vi "Visualize_Results_of_Filtering-1.vi"(7 "[IN] Number of event":i8=2, 8 "error IN":errorcluster, 9 "[IN] Localization Settings":T5 {"[IN] Image Type" items=["Grayscale (U8)", "Grayscale (I16)", "Grayscale (SGL)", "Complex (CSG)", "RGB (U32)", "HSL (U32)", "RGB (U64)", "Grayscale (U16)"]; "[IN] Particle Filter Setups"."Type of particle filter"."Measurement Parameter" items=["Center of Mass X", "Center of Mass Y", "First Pixel X", "First Pixel Y", "Bounding Rect Left", "Bounding Rect Top", "Bounding Rect Right", "Bounding Rect Bottom", "Max Feret Diameter Start X", "Max Feret Diameter Start Y", "Max Feret Diameter End X", "Max Feret Diameter End Y", "Max Horiz. Segment Length Left", "Max Horiz. Segment Length Right", "Max Horiz. Segment Length Row", "-", "Bounding Rect Width", "Bounding Rect Height", "Bounding Rect Diagonal", "Perimeter", "Convex Hull Perimeter", "Holes' Perimeter", "Max Feret Diameter", "Equivalent Ellipse Major Axis", "Equivalent Ellipse Minor Axis", "Equivalent Ellipse Minor Axis (Feret)", "Equivalent Rect Long Side", "Equivalent Rect Short Side", "Equivalent Rect Diagonal", "Equivalent Rect Short Side (Feret)", "Average Horiz. Segment Length", "Average Vert. Segment Length", "Hydraulic Radius", "Waddel Disk Diameter", "-", "Area", "Holes' Area", "Particle & Holes' Area", "Convex Hull Area", "Image Area", "-", "Number of Holes", "Number of Horiz. Segments", "Number of Vert. Segments", "-", "Orientation", "Max Feret Diameter Orientation", "-", "% Area/Image Area", "% Area/(Particle & Holes' Area)", "Ratio of Equivalent Ellipse Axes", "Ratio of Equivalent Rect Sides", "-", "Elongation Factor", "Compactness Factor", "Heywood Circularity Factor", "Type Factor", "-", "Sum X", "Sum Y", "Sum XX", "Sum XY", "Sum YY", "Sum XXX", "Sum XXY", "Sum XYY", "Sum YYY", "-", "Moment of Inertia XX", "Moment of Inertia XY", "Moment of Inertia YY", "Moment of Inertia XXX", "Moment of Inertia XXY", "Moment of Inertia XYY", "Moment of Inertia YYY", "Norm. Moment of Inertia XX", "Norm. Moment of Inertia XY", "Norm. Moment of Inertia YY", "Norm. Moment of Inertia XXX", "Norm. Moment of Inertia XXY", "Norm. Moment of Inertia XYY", "Norm. Moment of Inertia YYY", "Hu Moment 1", "Hu Moment 2", "Hu Moment 3", "Hu Moment 4", "Hu Moment 5", "Hu Moment 6", "Hu Moment 7"]}, 10 "# Frame":u32 max=499, 11 "[IN] Images Array":T1[](array[typedef])) -> (0 "error OUT":errorcluster, 2 "[OUT] LoG with Particles":T1, 3 "[OUT] Binarized Image":T1)   [LabVIEW 2017]
doc: "This subVI performs gamma correction and convolution of selected frame with the LoG"
uses:
  <vilib>/vision/Image Controls.llb/IMAQ Image.ctl
  <vilib>/vision/Avi.llb/IMAQ AVI2 Refnum.ctl
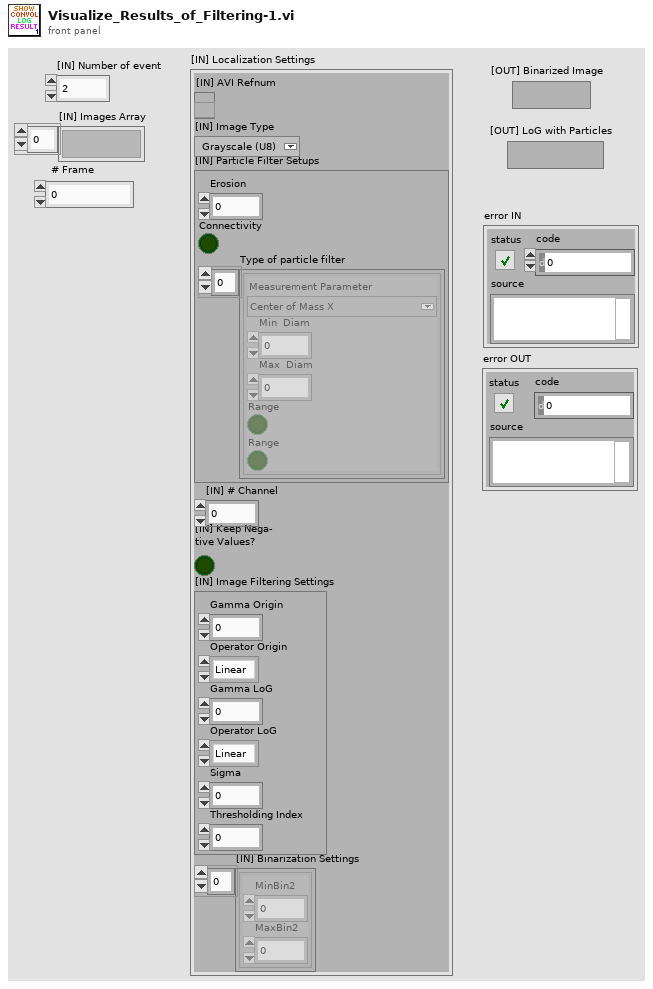
[diagram p1: front panel]
types:
  T1 = typedef "IMAQ Image.ctl" = refnum<image>
  T2 = typedef "IMAQ AVI2 Refnum.ctl" = refnum<k20>
  T3 = typedef "Image Type" = u32
  T4 = typedef "Particle Parameters" = i32
  T5 = cluster{"[IN] AVI Refnum":T2, "[IN] Image Type":T3, "[IN] Particle Filter Setups":cluster{"Erosion":i32, "Connectivity ":bool, "Type of particle filter":cluster{"Measurement Parameter":T4, "Min  Diam":dbl, "Max  Diam":dbl, "Range":bool, "Range":bool}[]}, "[IN] # Channel":u8, "[IN] Keep Nega-\ntive Values?":bool, "[IN] Image Filtering Settings":cluster{"Gamma Origin":sgl, "Operator Origin":enum32{"Linear", "Log", "Exp", "Square", "Square root", "Power X", "Power 1/X"}, "Gamma LoG":sgl, "Operator LoG":enum32{"Linear", "Log", "Exp", "Square", "Square root", "Power X", "Power 1/X"}, "Sigma":dbl, "Thresholding Index":i8}, "[IN] Binarization Settings":cluster{"MinBin2":sgl, "MaxBin2":sgl}[]}
  T6 = cluster{"Erosion":i32, "Connectivity ":bool, "Type of particle filter":cluster{"Measurement Parameter":T4, "Min  Diam":dbl, "Max  Diam":dbl, "Range":bool, "Range":bool}[]}
  T7 = cluster{"Gamma Origin":sgl, "Operator Origin":enum32{"Linear", "Log", "Exp", "Square", "Square root", "Power X", "Power 1/X"}, "Gamma LoG":sgl, "Operator LoG":enum32{"Linear", "Log", "Exp", "Square", "Square root", "Power X", "Power 1/X"}, "Sigma":dbl, "Thresholding Index":i8}
  T8 = cluster{"Area":dbl, "Number of Holes":dbl, "Bounding Rect":cluster{"Left":dbl, "Top":dbl, "Right":dbl, "Bottom":dbl}, "Center of Mass":cluster{"X":dbl, "Y":dbl}, "Orientation":dbl, "Dimensions":cluster{"Width":dbl, "Height":dbl}}[]
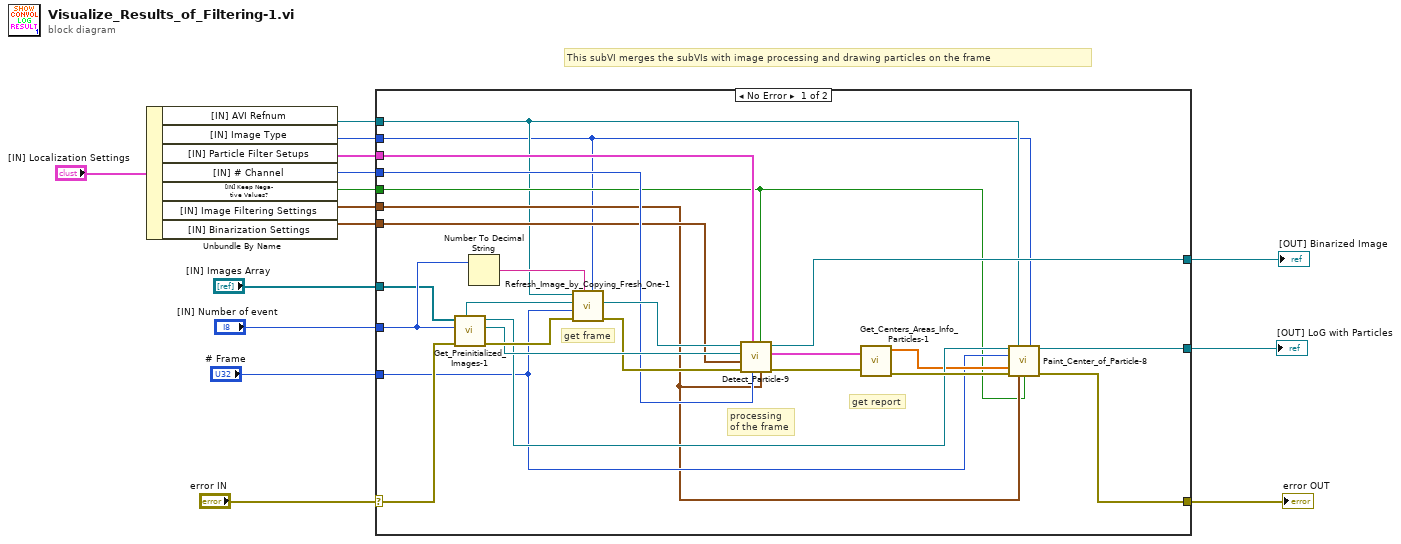
[diagram p0: block diagram]
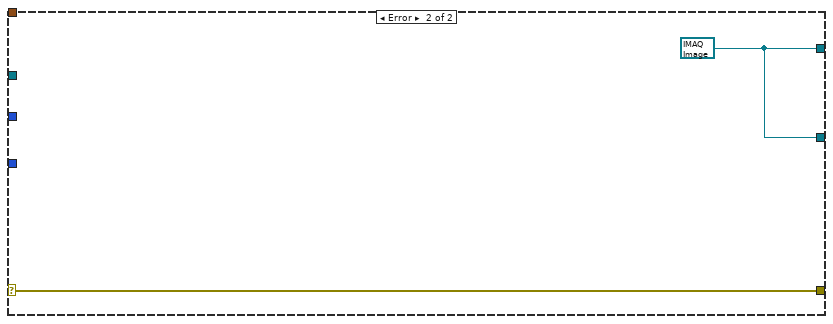
[diagram p2: hidden frame]
diagram:
  # "This subVI merges the subVIs with image processing and drawing particles on the frame"
  n1 = Unbundle By Name("[IN] Localization Settings") -> ("[IN] AVI Refnum"=w9:T2, "[IN] Image Type"=w8:T3, "[IN] Particle Filter Setups"=w7:T6, "[IN] # Channel"=w6:u8, "[IN] Keep Nega-\ntive Values?"=w5:bool, "[IN] Image Filtering Settings"=w4:T7, "[IN] Binarization Settings"=w3:cluster{"MinBin2":sgl, "MaxBin2":sgl}[])
  n2 = case shown="No Error" "error IN" {
    selector: "error IN" -> [w32 w42]
    tunnel: [w17 w42] -> w14
    tunnel: "[IN] Number of event" -> [w31 _]
    tunnel: "# Frame" -> [w22 _]
    tunnel: "[IN] Images Array" -> [w30 _]
    tunnel: w9 -> [w19 _]
    tunnel: w8 -> [w18 _]
    tunnel: w7 -> [w29 _]
    tunnel: w6 -> [w28 _]
    tunnel: w5 -> [w20 _]
    tunnel: w4 -> [w21 _]
    tunnel: w3 -> [w27 _]
    tunnel: [w26 w41] -> w2
    tunnel: [w16 w41] -> w1
    frame No Error {
      # "get report"
      # "processing\nof the frame"
      # "get frame"
      n3 = call "Get_Preinitialized_Images-1.vi"("error IN"=w32, "[IN] Number of event"=w31, "[IN] Images Array"=w30) -> ("error OUT"=w40:errorcluster, "[OUT] Processed Image #1"=w36:T1, "[OUT] Source Image #2"=w24:T1, "[OUT] Source Image #1"=w39:T1)  [unwired: 1 in, 1 out]
      n4 = Number To Decimal String(number=w31) -> (decimal integer string=w38:string)  [unwired: 1 in]
      n5 = call "Refresh_Image_by_Copying_Fresh_One-1.vi"("[IN] Image Type"=w18, "[IN] Unique ID\n(# of Event)"=w38, "error IN"=w40, "Frame Number"=w22, "[IN] Preinitialized Image"=w39, "[IN] AVI Refnum"=w19) -> ("error OUT"=w35:errorcluster, "[OUT] Frame"=w37:T1)  [unwired: 1 in, 1 out]
      n6 = call "Detect_Particle-9.vi"("[IN] Image Filtering Settings"=w21, "Keep Nega-\ntive Values?"=w20, "# Channel"=w28, "Particle Searching Settings"=w29, "error IN"=w35, "[IN] Binarization Settings"=w27, "[IN] Destination Image"=w36, "[IN] Frame"=w37) -> ("error OUT"=w33:errorcluster, "[OUT] Particle Reports (Pixels)"=w34:T8, "[OUT] Binarized Image"=w26:T1)  [unwired: 1 in]
      n7 = call "Get_Centers_Areas_Info_Particles-1.vi"("[IN] Particle Reports (Pixels)"=w34, "error in"=w33) -> ("[OUT] Array of X,Y"=w23:dbl[], "error out"=w25:errorcluster)  [unwired: 2 out]
      n8 = call "Paint_Center_of_Particle-8.vi"("[IN] Initialized Image"=w24, "[IN] AVI Refnum"=w19, "[IN] Image Type"=w18, "[IN] Frame Number"=w22, "[IN] Array of X,Y"=w23, "error IN"=w25, "[IN] Image Filtering Settings"=w21, "Keep Nega-\ntive Values?"=w20) -> ("[OUT] Image Dst"=w16:T1, "error OUT"=w17:errorcluster)  [unwired: 6 in]
    }
    frame Error {
      w41 = T1 refnum ("[OUT] Binarized Image")
    }
  }
  "error OUT" <- w14
  "[OUT] Binarized Image" <- w2
  "[OUT] LoG with Particles" <- w1
